vi "6-2.vi"() -> ()   [LabVIEW 2017]
uses:
  <vilib>/Waveform/WDTFileIO.llb/ Write Waveform to File.vi
  <vilib>/Waveform/WDTFileIO.llb/Read Waveform from File.vi
  <vilib>/measure/NI_MABase.lvlib
panel:
  out "波形图":waveform(dbl)(graph)
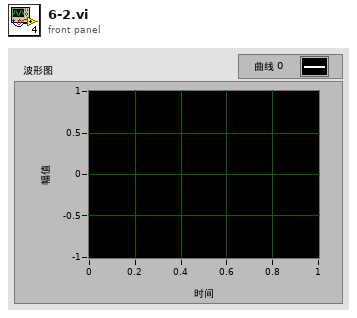
[diagram p1: front panel]
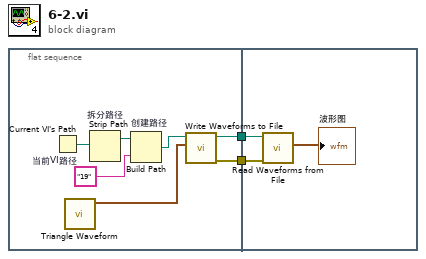
[diagram p0: block diagram]
diagram:
  n1 = flat-sequence {
    tunnel: [w4] -> w2
    tunnel: [w3] -> w1
    tunnel: w2 -> [w11]
    tunnel: w1 -> [w10]
    frame #0 {
      n2 = Current VI's Path "当前VI路径"() -> (path=w8:path)
      n3 = call <vilib>:"Triangle Waveform.vi"() -> ("signal out"=w6:waveform(dbl))  [unwired: 10 in, 1 out]
      n4 = Strip Path "拆分路径"(path=w8) -> (stripped path=w7:path)  [unwired: 1 out]
      n5 = Build Path "创建路径"(base path=w7, name or relative path="19" ("名称或相对路径")) -> (appended path=w9:path)
      n6 = call-poly <vilib>:"Write Waveforms to File.vi"("waveform"=w6, "file path (dialog if empty)"=w9) -> ("error out"=w3:errorcluster, "new file path (Not A Path if cancelled)"=w4:path)  [unwired: 8 in]
    }
    frame #1 {
      n7 = call-poly <vilib>:"Read Waveforms from File.vi"("error in (no error)"=w10, "file path (dialog if empty)"=w11) -> ("first waveform in record"=→"波形图":waveform(dbl))  [unwired: 4 in, 3 out]
    }
  }
